vi "Post Build Package Mods.vi"(8 "error in (no error)":errorcluster, 9 "Built package path":path, 11 "Project Root":path) -> (0 "error out":errorcluster)   [LabVIEW 2011]
uses:
  <userlib>/_OpenG.lib/file/file.llb/Strip Path Extension - Path__ogtk.vi
  <userlib>/_OpenG.lib/file/file.llb/File Exists - Scalar__ogtk.vi
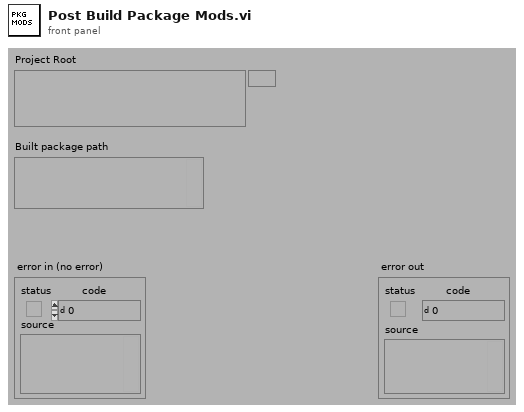
[diagram p1: front panel]
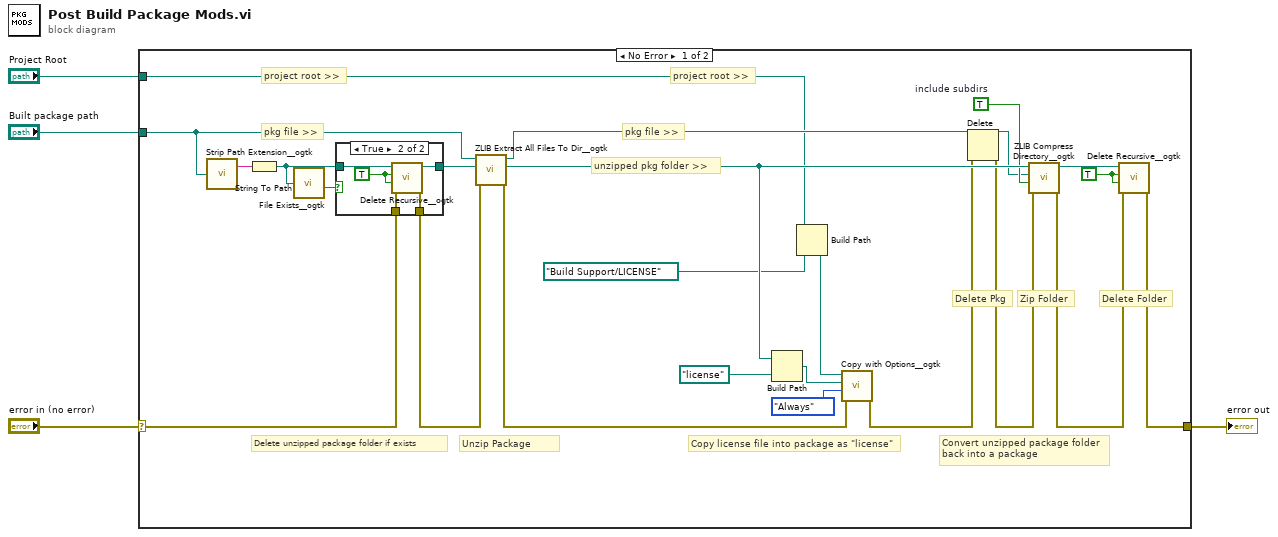
[diagram p0: block diagram]
diagram:
  n1 = case shown="No Error" "error in (no error)" {
    selector: "error in (no error)" -> [w25 w36]
    tunnel: [w11 w36] -> w3
    tunnel: "Built package path" -> [w28 _]
    tunnel: "Project Root" -> [w6 _]
    frame No Error {
      w14 = TRUE ("Recursive? (FALSE)")
      w19 = TRUE  # include subdirs
      # "project root >>"
      # "pkg file >>"
      # "project root >>"
      # "Delete Pkg"
      # "Zip Folder"
      # "Delete Folder"
      # "Convert unzipped package folder back into a package"
      # "Copy license file into package as \"license\""
      # "Delete unzipped package folder if exists"
      # "pkg file >>"
      # "unzipped pkg folder >>"
      # "Unzip Package"
      n2 = call-poly <userlib>:"Strip Path Extension__ogtk.vi"("path"=w28) -> ("root"=w27:string)  [unwired: 1 out]
      n3 = String To Path(string=w27) -> (path=w26:path)
      n4 = call-poly <userlib>:"File Exists__ogtk.vi"("file path"=w26) -> ("exists"=w22:bool)  [unwired: 6 in, 1 out]
      n5 = case shown="True" w22 {
        tunnel: w26 -> [w29 w35]
        tunnel: w25 -> [w30 w34]
        tunnel: [w30 w33] -> w23
        tunnel: [w29 w32] -> w24
        frame False {
        }
        frame True {
          w31 = TRUE ("Recursive? (FALSE)")
          n6 = call <userlib>:"Delete Recursive__ogtk.vi"("error in (no error)"=w34, "Ignore Read-Only? (FALSE)"=w31, "Recursive? (FALSE)"=w31, "Path"=w35) -> ("error out"=w33:errorcluster, "dup Path"=w32:path)  [unwired: 6 in]
        }
      }
      n7 = call <userlib>:"ZLIB Extract All Files To Dir__ogtk.vi"("error in (no error)"=w23, "root directory (archive name without ending)"=w24, "archive name (file dialog)"=w28) -> ("error out"=w10:errorcluster, "root directory out"=w20:path, "archive name out"=w18:path)  [unwired: 6 in]
      n8 = Build Path(base path=w20, name or relative path=path "license") -> (appended path=w9:path)
      n9 = Build Path(base path=w6, name or relative path=path "Build Support/LICENSE") -> (appended path=w7:path)
      n10 = call <userlib>:"Copy with Options__ogtk.vi"("error in (no error)"=w10, "Replace Mode (Never)"=enum16{"Never", "Always", "If Newer"}."Always", "target path"=w9, "source path"=w7) -> ("error out"=w16:errorcluster)  [unwired: 6 in, 1 out]
      n11 = Delete(path (use dialog)=w18, error in=w16) -> (deleted path=w17:path, error out=w15:errorcluster)  [unwired: 3 in, 1 out]
      n12 = call <userlib>:"ZLIB Compress Directory__ogtk.vi"("error in (no error)"=w15, "include subdirectories (F)"=w19, "archive name (root directory with .zip ending)"=w17, "root directory (file dialog)"=w20) -> ("error out"=w12:errorcluster, "root directory out"=w13:path)  [unwired: 5 in, 1 out]
      n13 = call <userlib>:"Delete Recursive__ogtk.vi"("error in (no error)"=w12, "Ignore Read-Only? (FALSE)"=w14, "Recursive? (FALSE)"=w14, "Path"=w13) -> ("error out"=w11:errorcluster)  [unwired: 6 in, 1 out]
    }
    frame Error {
    }
  }
  "error out" <- w3
